vi "myRIO-1900 Customized FPGA.vi"() -> ()   [LabVIEW 2013]
doc: "This VI contains the default FPGA personality in addition to code that filters data based on Frequency Selector and sends data to RT Main.vi through FIFO. Keeping the default personality allows you to continue using the myRIO APIs even after adding custom FPGA code."
uses:
  Sub VIs/Utilities/Start Boolean.ctl
  <vilib>/Platform/TimedLoop/XDataNode/timing_clust.ctl
  <vilib>/Platform/TimedLoop/XDataNode/nitl_modes.ctl
  <vilib>/Platform/TimedLoop/XDataNode/wakeup.ctl
  <vilib>/rvi/Emulation/niFpgaSctlEmulationGetInTimedLoop.vi
  <vilib>/rvi/Emulation/niFpgaEmulationReportErrorSimple.vi
  <vilib>/rvi/Emulation/niFpgaGetClockAttributes.vi
  <vilib>/rvi/Emulation/niFpgaCriticalErrorInLSC.vi
  <vilib>/rvi/eio/common/nirviEmuTemplateMethod_errors.vi
  <vilib>/rvi/eio/common/nirviEmuTemplatePropertyGet_noerrors.vi
  <vilib>/Platform/TimedLoop/XDataNode/XDataNode.xnode
  <vilib>/eio/EIONode/EIONode.xnode
  <vilib>/eio/EIOPropertyNode/EIOPropertyNode.xnode
  <vilib>/rvi/Analysis/measure/butterworth/XNode/niFpgaButterworthFilter.xnode
  <vilib>/Platform/TimedLoop/XDataNode/XDNodeRunTimeDep.lvlib
  <vilib>/rvi/eio/common/nirviEmuTemplatePropertyGet_errors.vi
  <vilib>/rvi/eio/common/nirviEmuTemplatePropertySet_errors.vi
  <vilib>/rvi/eio/common/nirviEmuTemplatePropertySet_noerrors.vi
panel:
  in  "Frequency Selector":T1(ring)
  out "ACC.SCALE.WGHT":u16
  out "SYS.ACC_SCALE.RDY":bool
  out "AO.SYS.STAT":bool
  out "AI.B_1.WGHT":u32
  out "AO.B_0.WGHT":u32
  out "AO.B_1.WGHT":u32
  out "AO.B_0.OFST":u32
  out "AO.B_1.OFST":u32
  out "AO.A_0.WGHT":u32
  out "AO.A_1.WGHT":u32
  out "AO.C_0.WGHT":u32
  out "AO.C_1.WGHT":u32
  out "AO.AudioOut_L.WGHT":u32
  out "AO.AudioOut_R.WGHT":u32
  out "AO.A_0.OFST":u32
  out "AO.C_0.OFST":u32
  out "AO.C_1.OFST":u32
  out "AO.AudioOut_L.OFST":u32
  out "AO.AudioOut_R.OFST":u32
  out "AO.A_1.OFST":u32
  out "SYS.AO_SCALE.RDY":bool
  out "SYS.AI_SCALE.RDY":bool
  out "AI.A_1.OFST":u32
  out "AI.A_2.OFST":u32
  out "AI.A_3.OFST":u32
  out "AI.B_0.OFST":u32
  out "AI.B_1.OFST":u32
  out "AI.B_2.OFST":u32
  out "AI.B_3.OFST":u32
  out "AI.C_0.OFST":u32
  out "AI.C_1.OFST":u32
  out "AI.AudioIn_L.OFST":u32
  out "AI.AudioIn_R.OFST":u32
  out "AI.A_0.OFST":u32
  out "AI.AudioIn_R.WGHT":u32
  out "AI.AudioIn_L.WGHT":u32
  out "AI.C_1.WGHT":u32
  out "AI.C_0.WGHT":u32
  out "AI.B_3.WGHT":u32
  out "AI.B_2.WGHT":u32
  out "AI.B_0.WGHT":u32
  out "AI.A_3.WGHT":u32
  out "AI.A_2.WGHT":u32
  out "AI.A_1.WGHT":u32
  out "AI.A_0.WGHT":u32
  out "DI.BTN":u8 format="%08b"
  in  "DO.LED3:0":u8 format="%04b"
  out "ACC.Z.VAL":u16
  out "SYS.ACC.RDY":bool
  out "ACC.Y.VAL":u16
  out "ACC.X.VAL":u16
  in  "AO.SYS.GO":T2
  in  "AO.AudioOut_L.VAL":i16
  in  "AO.AudioOut_R.VAL":i16
  out "AI.AudioIn_L.VAL":i16
  out "AI.AudioIn_R.VAL":i16
  in  "DIO.B_15:8.OUT":u8 format="%08b"
  in  "DIO.B_15:8.DIR":u8 format="%08b"
  out "DIO.B_15:8.IN":u8 format="%08b"
  in  "DIO.A_15:8.DIR":u8 format="%08b"
  in  "DIO.A_15:8.OUT":u8 format="%08b"
  out "DIO.A_15:8.IN":u8 format="%08b"
  in  "PWM.C_0.MAX":u16
  in  "PWM.C_0.CMP":u16
  out "PWM.C_0.CNTR":u16
  in  "PWM.C_0.CNFG":u8 format="%08b"
  in  "PWM.C_0.CS":u8
  in  "PWM.C_1.MAX":u16
  in  "PWM.C_1.CMP":u16
  out "PWM.C_1.CNTR":u16
  in  "PWM.C_1.CNFG":u8 format="%08b"
  in  "PWM.C_1.CS":u8
  out "ENC.C_1.STAT":u8 format="%08b"
  out "ENC.C_1.CNTR":u32
  in  "ENC.C_1.CNFG":u8 format="%08b"
  out "ENC.C_0.STAT":u8 format="%08b"
  out "ENC.C_0.CNTR":u32
  in  "ENC.C_0.CNFG":u8 format="%08b"
  in  "SYS.SELECTA":u8 format="%08b"
  in  "SYS.SELECTC":u8 format="%08b"
  in  "SYS.SELECTB":u8 format="%08b"
  in  "AO.C_1.VAL":u16
  in  "AO.C_0.VAL":u16
  out "AI.C_0.VAL":u16
  out "AI.C_1.VAL":u16
  in  "DIO.C_7:0.OUT":u8 format="%08b"
  in  "DIO.C_7:0.DIR":u8 format="%08b"
  out "DIO.C_7:0.IN":u8 format="%08b"
  in  "DIO.A_7:0.DIR":u8 format="%08b"
  in  "DIO.A_7:0.OUT":u8 format="%08b"
  out "DIO.A_7:0.IN":u8 format="%08b"
  in  "PWM.B_0.CMP":u16
  in  "PWM.B_0.MAX":u16
  out "PWM.B_0.CNTR":u16
  in  "PWM.B_0.CNFG":u8 format="%08b"
  in  "PWM.B_0.CS":u8
  in  "PWM.B_1.CMP":u16
  in  "PWM.B_1.MAX":u16
  out "PWM.B_1.CNTR":u16
  in  "PWM.B_1.CNFG":u8 format="%08b"
  in  "PWM.B_1.CS":u8
  in  "PWM.B_2.CMP":u16
  in  "PWM.B_2.MAX":u16
  out "PWM.B_2.CNTR":u16
  in  "PWM.B_2.CNFG":u8 format="%08b"
  in  "PWM.B_2.CS":u8
  out "SYS.RDY":bool
  out "SYS.AI.RDY":bool
  in  "I2C.B.GO":T2
  in  "I2C.A.GO":T2
  in  "I2C.A.CNFG":u8 format="%08b"
  in  "I2C.B.CNFG":u8 format="%08b"
  in  "I2C.A.DATO":u8
  out "I2C.A.DATI":u8
  in  "I2C.A.ADDR":u8 format="%08b"
  in  "I2C.A.CNTR":u8
  in  "I2C.B.DATO":u8
  out "I2C.B.DATI":u8
  in  "I2C.B.ADDR":u8 format="%08.0f"
  in  "I2C.B.CNTR":u8
  in  "I2C.A.CNTL":u8 format="%08b"
  out "I2C.A.STAT":u8 format="%08b"
  in  "I2C.B.CNTL":u8 format="%08b"
  out "I2C.B.STAT":u8 format="%08b"
  out "SPI.B.STAT":u8 format="%08b"
  in  "SPI.B.GO":T2
  out "SPI.A.STAT":u8 format="%08b"
  in  "SPI.A.GO":T2
  out "ENC.B.STAT":u8 format="%08b"
  out "ENC.A.STAT":u8 format="%08b"
  out "ENC.B.CNTR":u32
  out "ENC.A.CNTR":u32
  in  "ENC.B.CNFG":u8 format="%08b"
  in  "ENC.A.CNFG":u8 format="%08b"
  in  "SPI.B.DATO":u16
  out "SPI.B.DATI":u16
  in  "SPI.B.CNFG":u16 format="%016.0f"
  in  "SPI.B.CNT":u16
  in  "SPI.A.CNT":u16
  in  "SPI.A.CNFG":u16 format="%016b"
  out "SPI.A.DATI":u16
  in  "SPI.A.DATO":u16
  in  "PWM.A_0.MAX":u16
  in  "PWM.A_0.CMP":u16
  out "PWM.A_0.CNTR":u16
  in  "PWM.A_0.CNFG":u8 format="%08b"
  in  "PWM.A_0.CS":u8
  in  "PWM.A_1.CMP":u16
  in  "PWM.A_1.MAX":u16
  out "PWM.A_1.CNTR":u16
  in  "PWM.A_1.CNFG":u8 format="%08b"
  in  "PWM.A_1.CS":u8
  in  "PWM.A_2.CMP":u16
  in  "PWM.A_2.MAX":u16
  out "PWM.A_2.CNTR":u16
  in  "PWM.A_2.CNFG":u8 format="%08b"
  in  "PWM.A_2.CS":u8
  in  "DIO.B_7:0.OUT":u8 format="%08b"
  in  "DIO.B_7:0.DIR":u8 format="%08b"
  out "DIO.B_7:0.IN":u8 format="%08b"
  out "AI.A_0.VAL":u16
  out "AI.A_1.VAL":u16
  out "AI.A_2.VAL":u16
  out "AI.A_3.VAL":u16
  out "AI.B_0.VAL":u16
  out "AI.B_1.VAL":u16
  out "AI.B_2.VAL":u16
  out "AI.B_3.VAL":u16
  in  "AO.B_1.VAL":u16
  in  "AO.B_0.VAL":u16
  in  "AO.A_1.VAL":u16
  in  "AO.A_0.VAL":u16
  # "System"
  # "Onboard Devices"
  # "Connector A"
  # "Connector B"
  # "Connector C"
  # "Audio Connector"
  # "Accelerometer"
  # "Analog Input"
  # "Analog Output"
  # "Digital I/O"
  # "Counters / PWM"
  # "SPI Master"
  # "Analog Input"
  # "Analog Output"
  # "Digital I/O"
  # "Counters / PWM"
  # "SPI Master"
  # "Analog Input"
  # "Analog Output"
  # "Digital I/O"
  # "Counters / PWM"
  # "Analog Input"
  # "Encoders"
  # "Buttons & LEDs"
  # "I2C Master"
  # "I2C Master"
  # "Encoders"
  # "Encoders"
  # "Analog Output"
  # "IO Configuration"
  # "IO Configuration"
  # "IO Configuration"
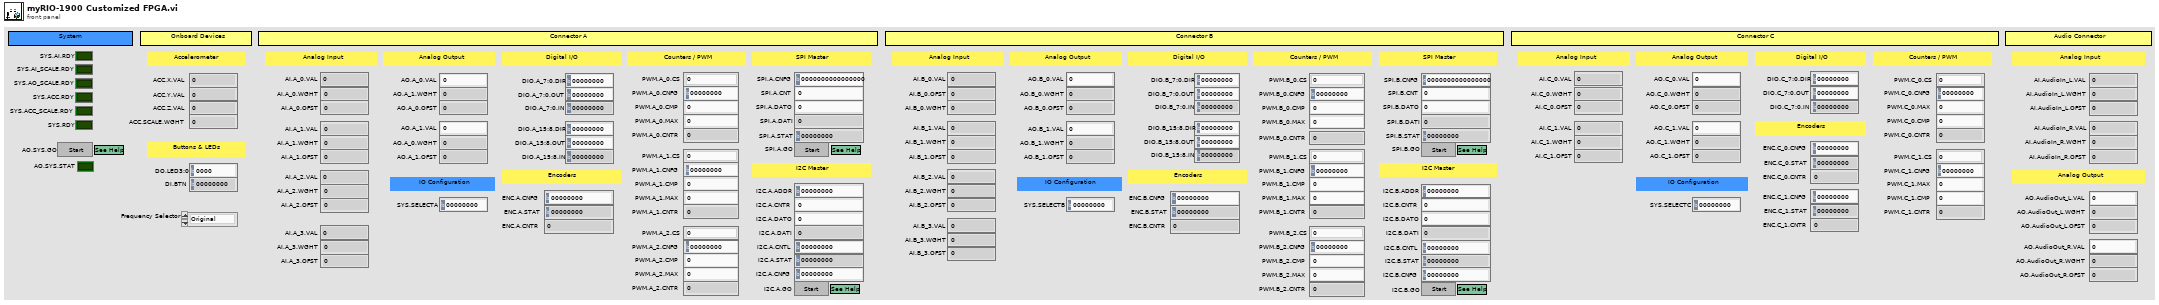
[diagram p1: front panel]
types:
  T1 = enum16{"Original", "< 500 Hz", "500 Hz - 1 kHz", "1 kHz - 2 kHz", "> 2 kHz"}
  T2 = typedef "Start Boolean.ctl" = bool
  T3 = typedef "XDNodeRunTimeDep.lvlib/timing_clust.ctl" = cluster{"Expected End [f-1]":u64, "Actual End [f-1]":u64, "Finished Late? [f-1]":bool, "Expected End [i-1]":u64, "Actual End [i-1]":u64, "Finished Late? [i-1]":bool, "Expected Start [i]":u64, "Actual Start [i]":u64, "Expected Start [f]":u64, "Actual Start [f]":u64, "Source Name":string, "Structure Name":string, "Period":i64, "Deadline":i64, "Offset":i64, "Start":i64, "Priority":i32, "Timeout":i32, "Mode":T4, "Wakeup Reason":T5, "Error":errorcluster, "Source Type":string, "Secondary Source Type":string, "Global End Time":u64, "Global Start Time":u64, "Frame Duration":u64, "Iteration Duration":u64, "Assigned CPU":i32, "I/O Scan Engine Mode":u32}
  T4 = typedef "XDNodeRunTimeDep.lvlib/nitl_modes.ctl" = enum32{"No Change", "Process missed periods, maintain original phase", "Discard missed periods, maintain original phase", "Process missed periods, ignore original phase", "Discard missed periods, ignore original phase"}
  T5 = typedef "XDNodeRunTimeDep.lvlib/wakeup.ctl" = enum32{"Normal", "Aborted", "Asynchronous wakeup", "Timing source error", "Timed loop error", "Timeout"}
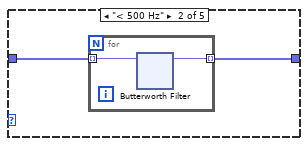
[diagram p3: hidden frame]
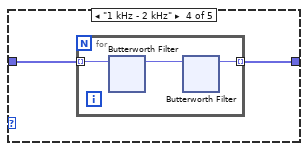
[diagram p4: hidden frame]
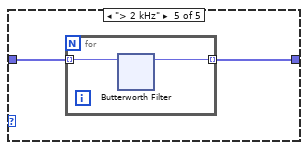
[diagram p5: hidden frame]
diagram:
  # "NOTE: The SYS.RDY boolean MUST exist and must become TRUE at some point otherwise the myRIO API will not function correctly."
  # "All DIO operations occur inside one single cycle timed loop (SCTL) since the IO is shared."
  # "The analog input scaling values are stored on the hardware. The RDY boolean should be checked before the values are used otherwise the analog input vlaues could be scaled incorrectly.\n\nAfter the first iteration of the while loop, all indicators have valid values."
  # "The analog output scaling values are stored on the hardware. The RDY boolean should be checked before the values are used otherwise the analog output vlaues could be scaled incorrectly.\n\nAfter the first iteration of the while loop, all indicators have valid values."
  # "The accelerometer nodes takes some time before the values can first be read (this is due to the time taken to read from the acceleromter). An iteration of the while loop will not complete until the accelerometer values have been read.\n\nAfter the first iteration of the while loop, all indicators have valid values."
  # "The onboard accelerometer has a range of +/- 8g which translates to 256 bits/g. The scaling weight is hardcoded in the FPGA to allow for future updates with minimal changes in the myRIO code. The RDY boolean should be checked before the values are used otherwise the analog output vlaues could be scaled incorrectly.\n\nAfter the first iteration of the while loop, all indicators have valid values."
  # "Onboard Accelerometer Scaling"
  # "Analog Output Scaling Constants"
  # "Analog Input Scaling Constants"
  # "Onboard Accelerometer"
  # "Onboard DIO"
  # "Connector B DIO"
  # "There is some delay between when the FPGA code starts and the analog inputs, accelerometer, and scaling values outputs are valid. If the host wants to ensure that there are valid values in theses registers it should wait for each subsystem to finish its initialization process. \n\nWhen all subsystems have finished initializinig, the SYS.RDY indicator will be true, which can be polled by the host to determine the status of the FPGA. Alternatively, the host can poll the individual SYS.xx.RDY indicators to determine the status of the individual subsystems.\n\nThis loop continues indefinitely, essentially making SYS.RDY a read-only register."
  # "The analog input nodes takes some time before the values can first be read (this is due to the time taken to setup the ADC and convert the first reading). An iteration of the while loop will not complete until all the analog input channels have been sampled.\n\nAfter the first iteration of the while loop, all indicators have valid values."
  # "Note: On some hardware a \"ghosting effect\" may occur on any unconnected AI channels. For example, if channel AI0 is connected and channels AI1 - AI7 are not connected the the value read at AI0 may be seen on indicators AI1 - AI7. This is common for hardware that use a multiplexed (MUXed) Analog-to-Digital converter (ADC) since the input analog signal is used to charge a capacitor which does not discharge before the unconnected channel is read.\n\n\"Ghosting\" effect can be hidden be using an mask register which will be used to decide when the indicator should be updated."
  # "The analog output nodes take some time before values are written to the pins. The GO and STAT registers are used to handshake between the FPGA and host. When the host wants the values to be written it sets the GO register to true. If the host reads the STAT register before setting GO, it can then wait for the STAT register value to invert which will tell the host that the output values have been written."
  # "Connector A DIO"
  # "Connector C  DIO"
  # "Host Synchronization"
  # "Analog Output"
  # "Analog Input"
  n1 = while {
    stop <- FALSE stop-if-true
    n2 = local read "SYS.ACC_SCALE.RDY"() -> (w10:bool)
    n3 = local read "SYS.AO_SCALE.RDY"() -> (w11:bool)
    n4 = local read "SYS.AI_SCALE.RDY"() -> (w12:bool)
    n5 = local read "SYS.ACC.RDY"() -> (w13:bool)
    n6 = local read "SYS.AI.RDY"() -> (w15:bool)
    n7 = Compound Arithmetic op=AND(w15, w13, w12, w11, w10) -> (→"SYS.RDY":bool)
  }
  n8 = while {
    i -> [w35]
    stop <- FALSE stop-if-true
    n9 = xnode "FPGA I/O Node"() -> ("ConnectorA/AI0"=→"AI.A_0.VAL":u16, "ConnectorA/AI1"=→"AI.A_1.VAL":u16, "ConnectorA/AI2"=→"AI.A_2.VAL":u16, "ConnectorA/AI3"=→"AI.A_3.VAL":u16, "ConnectorB/AI0"=→"AI.B_0.VAL":u16, "ConnectorB/AI1"=→"AI.B_1.VAL":u16, "ConnectorB/AI2"=→"AI.B_2.VAL":u16, "ConnectorB/AI3"=→"AI.B_3.VAL":u16, "ConnectorC/AI0"=w29:i16, "ConnectorC/AI1"=w28:i16, "AudioIn/Left"=w21:i16, "AudioIn/Right"=w20:i16)  [unwired: 12 in, 12 out]
    n10 = Greater Than 0?(x=w35) -> (x > 0?=→"SYS.AI.RDY":bool)
    n11 = To Unsigned Word Integer(number=w29) -> (unsigned 16bit integer=→"AI.C_0.VAL":u16)
    n12 = To Unsigned Word Integer(number=w28) -> (unsigned 16bit integer=→"AI.C_1.VAL":u16)
    n13 = To Fixed-Point(fixed-point type=fxp<+/-,32,17> 0.0 ("input data"), number=w21) -> (fixed-point=w26:fxp<+/-,32,17>)
    n14 = To Fixed-Point(fixed-point type=fxp<+/-,32,17> 0.0 ("input data"), number=w20) -> (fixed-point=w27:fxp<+/-,32,17>)
    n15 = Build Array(w26, w27) -> (w23:fxp<+/-,32,17>[])
    n16 = case shown="\"500 Hz - 1 kHz\"" "Frequency Selector" {
      tunnel: [w43 w45 w57 w80 w103] -> w18
      tunnel: w23 -> [w43 w44 w58 w81 w104]
      frame "Original", Default {
      }
      frame "< 500 Hz" {
        n17 = for {
          tunnel: [w47] -> w45 mode=indexing
          tunnel: w44 -> [w46] mode=indexing
          n18 = xnode "Butterworth Filter"("input data"=w46) -> ("output data"=w47:fxp<+/-,16,17>)  [unwired: 2 in, 1 out]
        }
      }
      frame "500 Hz - 1 kHz" {
        n19 = for {
          tunnel: w58 -> [w60] mode=indexing
          tunnel: [w59] -> w57 mode=indexing
          n20 = xnode "Butterworth Filter"("input data"=w60) -> ("output data"=w61:fxp<+/-,16,17>)  [unwired: 2 in, 1 out]
          n21 = xnode "Butterworth Filter"("input data"=w61) -> ("output data"=w59:fxp<+/-,16,17>)  [unwired: 2 in, 1 out]
        }
      }
      frame "1 kHz - 2 kHz" {
        n22 = for {
          tunnel: w81 -> [w83] mode=indexing
          tunnel: [w82] -> w80 mode=indexing
          n23 = xnode "Butterworth Filter"("input data"=w83) -> ("output data"=w84:fxp<+/-,16,17>)  [unwired: 2 in, 1 out]
          n24 = xnode "Butterworth Filter"("input data"=w84) -> ("output data"=w82:fxp<+/-,16,17>)  [unwired: 2 in, 1 out]
        }
      }
      frame "> 2 kHz" {
        n25 = for {
          tunnel: w104 -> [w106] mode=indexing
          tunnel: [w105] -> w103 mode=indexing
          n26 = xnode "Butterworth Filter"("input data"=w106) -> ("output data"=w105:fxp<+/-,16,17>)  [unwired: 2 in, 1 out]
        }
      }
    }
    n27 = To Word Integer(number=w18) -> (16bit integer=w19:i16[])
    n28 = Index Array(array=w19) -> (element #1=→"AI.AudioIn_L.VAL":i16, element #2=→"AI.AudioIn_R.VAL":i16)  [unwired: 2 in]
  }
  n29 = while {
    i -> [w118]
    stop <- FALSE stop-if-true
    n30 = Greater Than 0?(x=w118) -> (x > 0?=→"SYS.AI_SCALE.RDY":bool)
    n31 = xnode "FPGA I/O Property Node"("FPGA I/O In"=refnum<k21> "ConnectorA/AI0" ("FPGA I/O")) -> ("LSB Weight"=→"AI.A_0.WGHT":u32, "Offset"=w143:i32)  [unwired: 1 out]
    n32 = xnode "FPGA I/O Property Node"("FPGA I/O In"=refnum<k21> "ConnectorA/AI1" ("FPGA I/O")) -> ("LSB Weight"=→"AI.A_1.WGHT":u32, "Offset"=w131:i32)  [unwired: 1 out]
    n33 = xnode "FPGA I/O Property Node"("FPGA I/O In"=refnum<k21> "ConnectorA/AI2" ("FPGA I/O")) -> ("LSB Weight"=→"AI.A_2.WGHT":u32, "Offset"=w140:i32)  [unwired: 1 out]
    n34 = xnode "FPGA I/O Property Node"("FPGA I/O In"=refnum<k21> "ConnectorA/AI3" ("FPGA I/O")) -> ("LSB Weight"=→"AI.A_3.WGHT":u32, "Offset"=w139:i32)  [unwired: 1 out]
    n35 = xnode "FPGA I/O Property Node"("FPGA I/O In"=refnum<k21> "ConnectorB/AI0" ("FPGA I/O")) -> ("LSB Weight"=→"AI.B_0.WGHT":u32, "Offset"=w138:i32)  [unwired: 1 out]
    n36 = xnode "FPGA I/O Property Node"("FPGA I/O In"=refnum<k21> "ConnectorB/AI1" ("FPGA I/O")) -> ("LSB Weight"=→"AI.B_1.WGHT":u32, "Offset"=w137:i32)  [unwired: 1 out]
    n37 = xnode "FPGA I/O Property Node"("FPGA I/O In"=refnum<k21> "ConnectorB/AI2" ("FPGA I/O")) -> ("LSB Weight"=→"AI.B_2.WGHT":u32, "Offset"=w136:i32)  [unwired: 1 out]
    n38 = xnode "FPGA I/O Property Node"("FPGA I/O In"=refnum<k21> "ConnectorB/AI3" ("FPGA I/O")) -> ("LSB Weight"=→"AI.B_3.WGHT":u32, "Offset"=w135:i32)  [unwired: 1 out]
    n39 = xnode "FPGA I/O Property Node"("FPGA I/O In"=refnum<k21> "ConnectorC/AI0" ("FPGA I/O")) -> ("LSB Weight"=→"AI.C_0.WGHT":u32, "Offset"=w134:i32)  [unwired: 1 out]
    n40 = xnode "FPGA I/O Property Node"("FPGA I/O In"=refnum<k21> "ConnectorC/AI1" ("FPGA I/O")) -> ("LSB Weight"=→"AI.C_1.WGHT":u32, "Offset"=w133:i32)  [unwired: 1 out]
    n41 = xnode "FPGA I/O Property Node"("FPGA I/O In"=refnum<k21> "AudioIn/Left" ("FPGA I/O")) -> ("LSB Weight"=→"AI.AudioIn_L.WGHT":u32, "Offset"=w132:i32)  [unwired: 1 out]
    n42 = xnode "FPGA I/O Property Node"("FPGA I/O In"=refnum<k21> "AudioIn/Right" ("FPGA I/O")) -> ("LSB Weight"=→"AI.AudioIn_R.WGHT":u32, "Offset"=w142:i32)  [unwired: 1 out]
    n43 = To Unsigned Long Integer(number=w143) -> (unsigned 32bit integer=→"AI.A_0.OFST":u32)
    n44 = To Unsigned Long Integer(number=w131) -> (unsigned 32bit integer=→"AI.A_1.OFST":u32)
    n45 = To Unsigned Long Integer(number=w140) -> (unsigned 32bit integer=→"AI.A_2.OFST":u32)
    n46 = To Unsigned Long Integer(number=w139) -> (unsigned 32bit integer=→"AI.A_3.OFST":u32)
    n47 = To Unsigned Long Integer(number=w138) -> (unsigned 32bit integer=→"AI.B_0.OFST":u32)
    n48 = To Unsigned Long Integer(number=w137) -> (unsigned 32bit integer=→"AI.B_1.OFST":u32)
    n49 = To Unsigned Long Integer(number=w136) -> (unsigned 32bit integer=→"AI.B_2.OFST":u32)
    n50 = To Unsigned Long Integer(number=w135) -> (unsigned 32bit integer=→"AI.B_3.OFST":u32)
    n51 = To Unsigned Long Integer(number=w134) -> (unsigned 32bit integer=→"AI.C_0.OFST":u32)
    n52 = To Unsigned Long Integer(number=w133) -> (unsigned 32bit integer=→"AI.C_1.OFST":u32)
    n53 = To Unsigned Long Integer(number=w132) -> (unsigned 32bit integer=→"AI.AudioIn_L.OFST":u32)
    n54 = To Unsigned Long Integer(number=w142) -> (unsigned 32bit integer=→"AI.AudioIn_R.OFST":u32)
  }
  n55 = while {
    stop <- FALSE stop-if-true
    n56 = feedback #1(FALSE) -> (w169:bool)
    n57 = case shown="True" "AO.SYS.GO" {
      tunnel: "AO.C_0.VAL" -> [_ w189]
      tunnel: "AO.C_1.VAL" -> [_ w188]
      tunnel: "AO.A_0.VAL" -> [_ w193]
      tunnel: "AO.A_1.VAL" -> [_ w192]
      tunnel: "AO.B_0.VAL" -> [_ w191]
      tunnel: "AO.B_1.VAL" -> [_ w190]
      tunnel: "AO.AudioOut_L.VAL" -> [_ w182]
      tunnel: "AO.AudioOut_R.VAL" -> [_ w181]
      tunnel: w169 -> [w180 w185]
      tunnel: [w180 w183] -> w167
      frame False {
      }
      frame True {
        n58 = To Word Integer(number=w189) -> (16bit integer=w187:i16)
        n59 = To Word Integer(number=w188) -> (16bit integer=w186:i16)
        n60 = flat-sequence {
          tunnel: w193 -> [w202]
          tunnel: w192 -> [w201]
          tunnel: w191 -> [w200]
          tunnel: w190 -> [w199]
          tunnel: w187 -> [w198]
          tunnel: w186 -> [w197]
          tunnel: w182 -> [w196]
          tunnel: w181 -> [w195]
          tunnel: w185 -> [w194]
          tunnel: [w194] -> w184
          tunnel: w184 -> [w204]
          tunnel: [w203] -> w183
          frame #0 {
            n61 = xnode "FPGA I/O Node"("ConnectorA/AO0"=w202, "ConnectorA/AO1"=w201, "ConnectorB/AO0"=w200, "ConnectorB/AO1"=w199, "ConnectorC/AO0"=w198, "ConnectorC/AO1"=w197, "AudioOut/Left"=w196, "AudioOut/Right"=w195) -> ()  [unwired: 8 in, 8 out]
          }
          frame #1 {
            n62 = Not(x=w204) -> (.not. x?=w203:bool)
          }
        }
      }
    }
    "AO.SYS.STAT" <- w167
    n63 = feedback-in #1(w167) -> ()
  }
  n64 = while {
    i -> [w226]
    stop <- FALSE stop-if-true
    n65 = Greater Than 0?(x=w226) -> (x > 0?=→"SYS.AO_SCALE.RDY":bool)
    n66 = xnode "FPGA I/O Property Node"("FPGA I/O In"=refnum<k21> "ConnectorA/AO0" ("FPGA I/O")) -> ("LSB Weight"=→"AO.A_0.WGHT":u32, "Offset"=w237:i32)  [unwired: 1 out]
    n67 = xnode "FPGA I/O Property Node"("FPGA I/O In"=refnum<k21> "ConnectorA/AO1" ("FPGA I/O")) -> ("LSB Weight"=→"AO.A_1.WGHT":u32, "Offset"=w229:i32)  [unwired: 1 out]
    n68 = xnode "FPGA I/O Property Node"("FPGA I/O In"=refnum<k21> "ConnectorB/AO0" ("FPGA I/O")) -> ("LSB Weight"=→"AO.B_0.WGHT":u32, "Offset"=w235:i32)  [unwired: 1 out]
    n69 = xnode "FPGA I/O Property Node"("FPGA I/O In"=refnum<k21> "ConnectorB/AO1" ("FPGA I/O")) -> ("LSB Weight"=→"AO.B_1.WGHT":u32, "Offset"=w234:i32)  [unwired: 1 out]
    n70 = xnode "FPGA I/O Property Node"("FPGA I/O In"=refnum<k21> "ConnectorC/AO0" ("FPGA I/O")) -> ("LSB Weight"=→"AO.C_0.WGHT":u32, "Offset"=w233:i32)  [unwired: 1 out]
    n71 = xnode "FPGA I/O Property Node"("FPGA I/O In"=refnum<k21> "ConnectorC/AO1" ("FPGA I/O")) -> ("LSB Weight"=→"AO.C_1.WGHT":u32, "Offset"=w232:i32)  [unwired: 1 out]
    n72 = xnode "FPGA I/O Property Node"("FPGA I/O In"=refnum<k21> "AudioOut/Left" ("FPGA I/O")) -> ("LSB Weight"=→"AO.AudioOut_L.WGHT":u32, "Offset"=w231:i32)  [unwired: 1 out]
    n73 = xnode "FPGA I/O Property Node"("FPGA I/O In"=refnum<k21> "AudioOut/Right" ("FPGA I/O")) -> ("LSB Weight"=→"AO.AudioOut_R.WGHT":u32, "Offset"=w230:i32)  [unwired: 1 out]
    n74 = To Unsigned Long Integer(number=w237) -> (unsigned 32bit integer=→"AO.A_0.OFST":u32)
    n75 = To Unsigned Long Integer(number=w229) -> (unsigned 32bit integer=→"AO.A_1.OFST":u32)
    n76 = To Unsigned Long Integer(number=w235) -> (unsigned 32bit integer=→"AO.B_0.OFST":u32)
    n77 = To Unsigned Long Integer(number=w234) -> (unsigned 32bit integer=→"AO.B_1.OFST":u32)
    n78 = To Unsigned Long Integer(number=w233) -> (unsigned 32bit integer=→"AO.C_0.OFST":u32)
    n79 = To Unsigned Long Integer(number=w232) -> (unsigned 32bit integer=→"AO.C_1.OFST":u32)
    n80 = To Unsigned Long Integer(number=w231) -> (unsigned 32bit integer=→"AO.AudioOut_L.OFST":u32)
    n81 = To Unsigned Long Integer(number=w230) -> (unsigned 32bit integer=→"AO.AudioOut_R.OFST":u32)
  }
  n82 = node-c288() -> (w2:T3)  [unwired: 1 in]
  n83 = timed-loop {
    timing: w2 -> [_]
    timing-out: [_] -> w1
    stop <- _ stop-if-true
    n84 = xnode "FPGA I/O Node"() -> ("Button0"=w248:bool)  [unwired: 1 in, 1 out]
    n85 = Number To Boolean Array(number="DO.LED3:0") -> (Boolean array=w244:bool[])
    n86 = Build Array(w248) -> (w247:bool[])
    n87 = Index Array(array=w244) -> (element #1=w243:bool, element #2=w242:bool, element #3=w241:bool, element #4=w240:bool)  [unwired: 4 in]
    n88 = Boolean Array To Number(Boolean array=w247) -> (number=→"DI.BTN":u8)
    n89 = xnode "FPGA I/O Node"("LED0"=w243, "LED1"=w242, "LED2"=w241, "LED3"=w240) -> ()  [unwired: 4 in, 4 out]
  }
  n90 = while {
    i -> [w255]
    stop <- FALSE stop-if-true
    n91 = xnode "FPGA I/O Node"() -> ("AccelerationX"=w258:i16, "AccelerationY"=w257:i16, "AccelerationZ"=w256:i16)  [unwired: 3 in, 3 out]
    n92 = Greater Than 0?(x=w255) -> (x > 0?=→"SYS.ACC.RDY":bool)
    n93 = To Unsigned Word Integer(number=w258) -> (unsigned 16bit integer=→"ACC.X.VAL":u16)
    n94 = To Unsigned Word Integer(number=w257) -> (unsigned 16bit integer=→"ACC.Y.VAL":u16)
    n95 = To Unsigned Word Integer(number=w256) -> (unsigned 16bit integer=→"ACC.Z.VAL":u16)
  }
  n96 = while {
    i -> [w262]
    stop <- FALSE stop-if-true
    # "The onboard accelerometer has a range of +/-8g which translates to 256 bits / g. The scaling weight is hardcoded in the FPGA to"
    n97 = Greater Than 0?(x=w262) -> (x > 0?=→"SYS.ACC_SCALE.RDY":bool)
    "ACC.SCALE.WGHT" <- u16 256 ("ACC.SCALE.WGHT")
  }
  n98 = node-c288(w1) -> ()
  n99 = node-c288() -> (w6:T3)  [unwired: 1 in]
  n100 = timed-loop {
    timing: w6 -> [_]
    timing-out: [_] -> w5
    stop <- _ stop-if-true
    # "DIO / Encoder"
    # "DIO / I2C Master"
    # "DIO / PWM"
    # "DIO"
    # "DIO"
    # "DIO/ SPI Master"
    n101 = call "Split HDC Bank1 DIO.vi"("IN 7:0"="DIO.A_7:0.OUT") -> ("OUT 3:0"=w351:fxp<+,4,4>, "OUT 4"=w264:bool, "OUT 7:5"=w348:fxp<+,3,3>)
    n102 = call "Split HDC Bank1 DIO.vi"("IN 7:0"="DIO.A_7:0.DIR") -> ("OUT 3:0"=w350:fxp<+,4,4>, "OUT 4"=w349:bool, "OUT 7:5"=w347:fxp<+,3,3>)
    n103 = call "Split HDC Function Select.vi"("IN 7:0"="SYS.SELECTA") -> ("OUT 1:0"=w285:fxp<+,2,2>, "OUT 7"=w280:bool, "OUT 2"=w284:bool, "OUT 3"=w283:bool, "OUT 4"=w282:bool, "OUT 5"=w281:bool)
    n104 = call "DIO 4-bit.vi"("DIO0 Refnum"=refnum<k21> "ConnectorA/DIO0", "DIO1 Refnum"=refnum<k21> "ConnectorA/DIO1", "DIO2 Refnum"=refnum<k21> "ConnectorA/DIO2", "DIR 3:0"=w350, "OUT 3:0"=w351, "DIO3 Refnum"=refnum<k21> "ConnectorA/DIO3") -> ("IN 3:0"=w322:fxp<+,4,4>)  [unwired: 5 in]
    n105 = call "DIO 1-bit.vi"("DIR"=w349, "OUT"=w264, "DIO Refnum"=refnum<k21> "ConnectorA/DIO4") -> ("IN"=w321:bool)  [unwired: 8 in]
    n106 = call "DIO_SPI.vi"("DIO.2:0.OUT"=w348, "DIO.2:0.DIR"=w347, "SPI.CNT"="SPI.A.CNT", "SPI.CNFG"="SPI.A.CNFG", "SPI.DATO"="SPI.A.DATO", "SPI.GO"="SPI.A.GO", "DIO.2/SPI.MOSI Refnum"=refnum<k21> "ConnectorA/DIO7" ("DIO.2/SPI.SCLK"), "SELECT.1:0"=w285, "DIO.1/SPI.MISO Refnum"=refnum<k21> "ConnectorA/DIO6" ("DIO.1/SPI.MOSI"), "DIO.0/SPI.SCLK Refnum"=refnum<k21> "ConnectorA/DIO5" ("DIO.0/SPI.MISO")) -> ("DIO.2:0.IN"=w320:fxp<+,3,3>, "SPI.DATI"=→"SPI.A.DATI":u16, "SPI.STAT"=→"SPI.A.STAT":u8)  [unwired: 7 in]
    n107 = call "Join HDC Bank1 DIO.vi"("IN 7:5"=w320, "IN 4"=w321, "IN 3:0"=w322) -> ("OUT 7:0"=→"DIO.A_7:0.IN":u8)
    n108 = call "Split HDC Bank2 DIO.vi"("IN 7:0"="DIO.A_15:8.OUT") -> ("OUT 5"=w266:bool, "OUT 7:6"=w290:fxp<+,2,2>, "OUT 4:3"=w268:fxp<+,2,2>, "OUT 2"=w270:bool, "OUT 0"=w274:bool, "OUT 1"=w273:bool)  [unwired: 2 in]
    n109 = call "Split HDC Bank2 DIO.vi"("IN 7:0"="DIO.A_15:8.DIR") -> ("OUT 5"=w265:bool, "OUT 7:6"=w289:fxp<+,2,2>, "OUT 4:3"=w267:fxp<+,2,2>, "OUT 2"=w269:bool, "OUT 0"=w272:bool, "OUT 1"=w271:bool)  [unwired: 2 in]
    n110 = call "DIO_PWM.vi"("DIO.OUT"=w274, "DIO.DIR"=w272, "PWM.CS"="PWM.A_0.CS", "PWM.CNFG"="PWM.A_0.CNFG", "PWM.CMP"="PWM.A_0.CMP", "PWM.MAX"="PWM.A_0.MAX", "DIO/PWM"=refnum<k21> "ConnectorA/DIO8", "SELECT"=w284) -> ("DIO.IN"=w279:bool, "PWM.CNTR"=→"PWM.A_0.CNTR":u16)  [unwired: 10 in]
    n111 = call "DIO_PWM.vi"("DIO.OUT"=w273, "DIO.DIR"=w271, "PWM.CS"="PWM.A_1.CS", "PWM.CNFG"="PWM.A_1.CNFG", "PWM.CMP"="PWM.A_1.CMP", "PWM.MAX"="PWM.A_1.MAX", "DIO/PWM"=refnum<k21> "ConnectorA/DIO9", "SELECT"=w283) -> ("DIO.IN"=w278:bool, "PWM.CNTR"=→"PWM.A_1.CNTR":u16)  [unwired: 10 in]
    n112 = call "DIO_PWM.vi"("DIO.OUT"=w270, "DIO.DIR"=w269, "PWM.CS"="PWM.A_2.CS", "PWM.CNFG"="PWM.A_2.CNFG", "PWM.CMP"="PWM.A_2.CMP", "PWM.MAX"="PWM.A_2.MAX", "DIO/PWM"=refnum<k21> "ConnectorA/DIO10", "SELECT"=w282) -> ("DIO.IN"=w277:bool, "PWM.CNTR"=→"PWM.A_2.CNTR":u16)  [unwired: 10 in]
    n113 = call "DIO_Encoder.vi"("DIO.1:0.OUT"=w268, "DIO.1:0.DIR"=w267, "QE.CNFG"="ENC.A.CNFG", "DIO.1/QE.B"=refnum<k21> "ConnectorA/DIO12", "SELECT"=w281, "DIO.0/QE.A"=refnum<k21> "ConnectorA/DIO11") -> ("DIO.1:0.IN"=w276:fxp<+,2,2>, "QE.CNTR"=→"ENC.A.CNTR":u32, "QE.STAT"=→"ENC.A.STAT":u8)  [unwired: 11 in]
    n114 = call "DIO 1-bit.vi"("DIR"=w265, "OUT"=w266, "DIO Refnum"=refnum<k21> "ConnectorA/DIO13") -> ("IN"=w275:bool)  [unwired: 8 in]
    n115 = call "DIO_I2C.vi"("DIO.1:0.OUT"=w290, "DIO.1:0.DIR"=w289, "I2C.CNFG"="I2C.A.CNFG", "I2C.CNTL"="I2C.A.CNTL", "I2C.ADDR"="I2C.A.ADDR", "I2C.DATO"="I2C.A.DATO", "DIO.1/I2C.SDA"=refnum<k21> "ConnectorA/DIO15" ("DIO.1/I2C.SCL"), "I2C.CNTR"="I2C.A.CNTR", "DIO.0/I2C.SCL"=refnum<k21> "ConnectorA/DIO14" ("DIO.0/I2C.SDA"), "Execute?"="I2C.A.GO", "SELECT"=w280) -> ("DIO.1:0.IN"=w287:fxp<+,2,2>, "I2C.DATI"=→"I2C.A.DATI":u8, "I2C.STAT"=→"I2C.A.STAT":u8)  [unwired: 6 in]
    n116 = call "Join HDC Bank2 DIO.vi"("IN 7:6"=w287, "IN 5"=w275, "IN 4:3"=w276, "IN 0"=w279, "IN 2"=w277, "IN 1"=w278) -> ("OUT 7:0"=→"DIO.A_15:8.IN":u8)  [unwired: 4 in]
  }
  n117 = node-c288(w5) -> ()
  n118 = node-c288() -> (w4:T3)  [unwired: 1 in]
  n119 = timed-loop {
    timing: w4 -> [_]
    timing-out: [_] -> w3
    stop <- _ stop-if-true
    # "DIO / Encoder"
    # "DIO / I2C Master"
    # "DIO / PWM"
    # "DIO"
    # "DIO"
    # "DIO/ SPI Master"
    n120 = call "Split HDC Bank1 DIO.vi"("IN 7:0"="DIO.B_7:0.OUT") -> ("OUT 3:0"=w441:fxp<+,4,4>, "OUT 4"=w439:bool, "OUT 7:5"=w437:fxp<+,3,3>)
    n121 = call "Split HDC Bank1 DIO.vi"("IN 7:0"="DIO.B_7:0.DIR") -> ("OUT 3:0"=w440:fxp<+,4,4>, "OUT 4"=w438:bool, "OUT 7:5"=w436:fxp<+,3,3>)
    n122 = call "Split HDC Function Select.vi"("IN 7:0"="SYS.SELECTB") -> ("OUT 1:0"=w413:fxp<+,2,2>, "OUT 7"=w408:bool, "OUT 2"=w412:bool, "OUT 3"=w411:bool, "OUT 4"=w410:bool, "OUT 5"=w409:bool)
    n123 = call "DIO 4-bit.vi"("DIO0 Refnum"=refnum<k21> "ConnectorB/DIO0", "DIO1 Refnum"=refnum<k21> "ConnectorB/DIO1", "DIO2 Refnum"=refnum<k21> "ConnectorB/DIO2", "DIR 3:0"=w440, "OUT 3:0"=w441, "DIO3 Refnum"=refnum<k21> "ConnectorB/DIO3") -> ("IN 3:0"=w419:fxp<+,4,4>)  [unwired: 5 in]
    n124 = call "DIO 1-bit.vi"("DIR"=w438, "OUT"=w439, "DIO Refnum"=refnum<k21> "ConnectorB/DIO4") -> ("IN"=w418:bool)  [unwired: 8 in]
    n125 = call "DIO_SPI.vi"("DIO.2:0.OUT"=w437, "DIO.2:0.DIR"=w436, "SPI.CNT"="SPI.B.CNT", "SPI.CNFG"="SPI.B.CNFG", "SPI.DATO"="SPI.B.DATO", "SPI.GO"="SPI.B.GO", "DIO.2/SPI.MOSI Refnum"=refnum<k21> "ConnectorB/DIO7" ("DIO.2/SPI.SCLK"), "SELECT.1:0"=w413, "DIO.1/SPI.MISO Refnum"=refnum<k21> "ConnectorB/DIO6" ("DIO.1/SPI.MOSI"), "DIO.0/SPI.SCLK Refnum"=refnum<k21> "ConnectorB/DIO5" ("DIO.0/SPI.MISO")) -> ("DIO.2:0.IN"=w417:fxp<+,3,3>, "SPI.DATI"=→"SPI.B.DATI":u16, "SPI.STAT"=→"SPI.B.STAT":u8)  [unwired: 7 in]
    n126 = call "Join HDC Bank1 DIO.vi"("IN 7:5"=w417, "IN 4"=w418, "IN 3:0"=w419) -> ("OUT 7:0"=→"DIO.B_7:0.IN":u8)
    n127 = call "Split HDC Bank2 DIO.vi"("IN 7:0"="DIO.B_15:8.OUT") -> ("OUT 5"=w364:bool, "OUT 7:6"=w416:fxp<+,2,2>, "OUT 4:3"=w365:fxp<+,2,2>, "OUT 2"=w366:bool, "OUT 0"=w368:bool, "OUT 1"=w367:bool)  [unwired: 2 in]
    n128 = call "Split HDC Bank2 DIO.vi"("IN 7:0"="DIO.B_15:8.DIR") -> ("OUT 5"=w359:bool, "OUT 7:6"=w415:fxp<+,2,2>, "OUT 4:3"=w360:fxp<+,2,2>, "OUT 2"=w361:bool, "OUT 0"=w363:bool, "OUT 1"=w362:bool)  [unwired: 2 in]
    n129 = call "DIO_PWM.vi"("DIO.OUT"=w368, "DIO.DIR"=w363, "PWM.CS"="PWM.B_0.CS", "PWM.CNFG"="PWM.B_0.CNFG", "PWM.CMP"="PWM.B_0.CMP", "PWM.MAX"="PWM.B_0.MAX", "DIO/PWM"=refnum<k21> "ConnectorB/DIO8", "SELECT"=w412) -> ("DIO.IN"=w358:bool, "PWM.CNTR"=→"PWM.B_0.CNTR":u16)  [unwired: 10 in]
    n130 = call "DIO_PWM.vi"("DIO.OUT"=w367, "DIO.DIR"=w362, "PWM.CS"="PWM.B_1.CS", "PWM.CNFG"="PWM.B_1.CNFG", "PWM.CMP"="PWM.B_1.CMP", "PWM.MAX"="PWM.B_1.MAX", "DIO/PWM"=refnum<k21> "ConnectorB/DIO9", "SELECT"=w411) -> ("DIO.IN"=w357:bool, "PWM.CNTR"=→"PWM.B_1.CNTR":u16)  [unwired: 10 in]
    n131 = call "DIO_PWM.vi"("DIO.OUT"=w366, "DIO.DIR"=w361, "PWM.CS"="PWM.B_2.CS", "PWM.CNFG"="PWM.B_2.CNFG", "PWM.CMP"="PWM.B_2.CMP", "PWM.MAX"="PWM.B_2.MAX", "DIO/PWM"=refnum<k21> "ConnectorB/DIO10", "SELECT"=w410) -> ("DIO.IN"=w356:bool, "PWM.CNTR"=→"PWM.B_2.CNTR":u16)  [unwired: 10 in]
    n132 = call "DIO_Encoder.vi"("DIO.1:0.OUT"=w365, "DIO.1:0.DIR"=w360, "QE.CNFG"="ENC.B.CNFG", "DIO.1/QE.B"=refnum<k21> "ConnectorB/DIO12", "SELECT"=w409, "DIO.0/QE.A"=refnum<k21> "ConnectorB/DIO11") -> ("DIO.1:0.IN"=w355:fxp<+,2,2>, "QE.CNTR"=→"ENC.B.CNTR":u32, "QE.STAT"=→"ENC.B.STAT":u8)  [unwired: 11 in]
    n133 = call "DIO 1-bit.vi"("DIR"=w359, "OUT"=w364, "DIO Refnum"=refnum<k21> "ConnectorB/DIO13") -> ("IN"=w354:bool)  [unwired: 8 in]
    n134 = call "DIO_I2C.vi"("DIO.1:0.OUT"=w416, "DIO.1:0.DIR"=w415, "I2C.CNFG"="I2C.B.CNFG", "I2C.CNTL"="I2C.B.CNTL", "I2C.ADDR"="I2C.B.ADDR", "I2C.DATO"="I2C.B.DATO", "DIO.1/I2C.SDA"=refnum<k21> "ConnectorB/DIO15" ("DIO.1/I2C.SCL"), "I2C.CNTR"="I2C.B.CNTR", "DIO.0/I2C.SCL"=refnum<k21> "ConnectorB/DIO14" ("DIO.0/I2C.SDA"), "Execute?"="I2C.B.GO", "SELECT"=w408) -> ("DIO.1:0.IN"=w414:fxp<+,2,2>, "I2C.DATI"=→"I2C.B.DATI":u8, "I2C.STAT"=→"I2C.B.STAT":u8)  [unwired: 6 in]
    n135 = call "Join HDC Bank2 DIO.vi"("IN 7:6"=w414, "IN 5"=w354, "IN 4:3"=w355, "IN 0"=w358, "IN 2"=w356, "IN 1"=w357) -> ("OUT 7:0"=→"DIO.B_15:8.IN":u8)  [unwired: 4 in]
  }
  n136 = node-c288(w3) -> ()
  n137 = node-c288() -> (w8:T3)  [unwired: 1 in]
  n138 = timed-loop {
    timing: w8 -> [_]
    timing-out: [_] -> w7
    stop <- _ stop-if-true
    n139 = call "Split myDAQ DIO.vi"("IN 7:0"="DIO.C_7:0.OUT") -> ("OUT 2, OUT0"=w462:fxp<+,2,2>, "OUT 1"=w461:bool, "OUT 3"=w460:bool, "OUT 7"=w457:bool, "OUT 6, OUT 4"=w459:fxp<+,2,2>, "OUT 5"=w458:bool)  [unwired: 4 in]
    n140 = call "Split myDAQ DIO.vi"("IN 7:0"="DIO.C_7:0.DIR") -> ("OUT 2, OUT0"=w456:fxp<+,2,2>, "OUT 1"=w455:bool, "OUT 3"=w454:bool, "OUT 7"=w451:bool, "OUT 6, OUT 4"=w453:fxp<+,2,2>, "OUT 5"=w452:bool)  [unwired: 4 in]
    n141 = call "Split myDAQ Function Select.vi"("IN 7:0"="SYS.SELECTC") -> ("OUT 0"=w468:bool, "OUT 1"=w467:bool, "OUT 2"=w466:bool, "OUT 3"=w465:bool)  [unwired: 2 in]
    n142 = call "DIO_Encoder.vi"("DIO.1:0.OUT"=w462, "DIO.1:0.DIR"=w456, "QE.CNFG"="ENC.C_0.CNFG", "DIO.1/QE.B"=refnum<k21> "ConnectorC/DIO2", "SELECT"=w468, "DIO.0/QE.A"=refnum<k21> "ConnectorC/DIO0") -> ("DIO.1:0.IN"=w449:fxp<+,2,2>, "QE.CNTR"=→"ENC.C_0.CNTR":u32, "QE.STAT"=→"ENC.C_0.STAT":u8)  [unwired: 11 in]
    n143 = call "DIO 1-bit.vi"("DIR"=w455, "OUT"=w461, "DIO Refnum"=refnum<k21> "ConnectorC/DIO1") -> ("IN"=w448:bool)  [unwired: 8 in]
    n144 = call "DIO_PWM.vi"("DIO.OUT"=w460, "DIO.DIR"=w454, "PWM.CS"="PWM.C_0.CS", "PWM.CNFG"="PWM.C_0.CNFG", "PWM.CMP"="PWM.C_0.CMP", "PWM.MAX"="PWM.C_0.MAX", "DIO/PWM"=refnum<k21> "ConnectorC/DIO3", "SELECT"=w467) -> ("DIO.IN"=w447:bool, "PWM.CNTR"=→"PWM.C_0.CNTR":u16)  [unwired: 10 in]
    n145 = call "DIO_Encoder.vi"("DIO.1:0.OUT"=w459, "DIO.1:0.DIR"=w453, "QE.CNFG"="ENC.C_1.CNFG", "DIO.1/QE.B"=refnum<k21> "ConnectorC/DIO6", "SELECT"=w466, "DIO.0/QE.A"=refnum<k21> "ConnectorC/DIO4") -> ("DIO.1:0.IN"=w446:fxp<+,2,2>, "QE.CNTR"=→"ENC.C_1.CNTR":u32, "QE.STAT"=→"ENC.C_1.STAT":u8)  [unwired: 11 in]
    n146 = call "DIO 1-bit.vi"("DIR"=w452, "OUT"=w458, "DIO Refnum"=refnum<k21> "ConnectorC/DIO5") -> ("IN"=w445:bool)  [unwired: 8 in]
    n147 = call "DIO_PWM.vi"("DIO.OUT"=w457, "DIO.DIR"=w451, "PWM.CS"="PWM.C_1.CS", "PWM.CNFG"="PWM.C_1.CNFG", "PWM.CMP"="PWM.C_1.CMP", "PWM.MAX"="PWM.C_1.MAX", "DIO/PWM"=refnum<k21> "ConnectorC/DIO7", "SELECT"=w465) -> ("DIO.IN"=w444:bool, "PWM.CNTR"=→"PWM.C_1.CNTR":u16)  [unwired: 10 in]
    n148 = call "Join myDAQ DIO.vi"("IN 7"=w444, "IN 5"=w445, "IN 6, IN 4"=w446, "IN 2, IN 0"=w449, "IN 3"=w447, "IN 1"=w448) -> ("IN 7:0"=→"DIO.C_7:0.IN":u8)  [unwired: 4 in]
  }
  n149 = node-c288(w7) -> ()
